vi "Set and Get Col Head String.vi"(7 "Mode":T1, 8 "错误输入":errorcluster, 10 "ColHdr Out In":string, 11 "Listbox Ref":refnum<vi>) -> (0 "错误输出":errorcluster, 2 "ColHdr Out":string, 3 "Dup Listbox Ref":refnum<vi>)   [LabVIEW 2012, in "Listbox Tool.lvlib"]
uses:
  Listbox Tool.lvlib
  Custom Type/Read and Write Mode.ctl
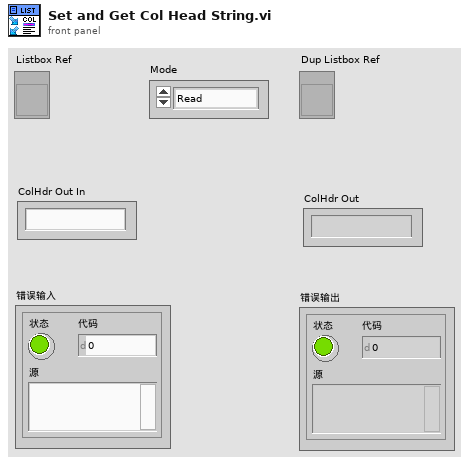
[diagram p1: front panel]
types:
  T1 = typedef "Listbox Tool.lvlib/Read and Write Mode.ctl" = enum16{"Read", "Write"}
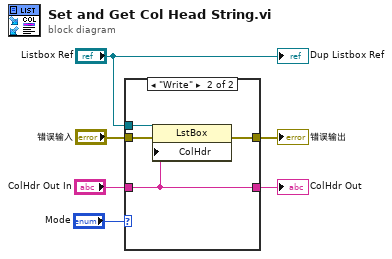
[diagram p0: block diagram]
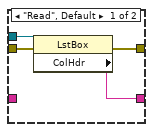
[diagram p2: hidden frame]
diagram:
  n1 = case shown="\"Write\"" "Mode" {
    tunnel: "ColHdr Out In" -> [_ w14]
    tunnel: [w10 w14] -> w4
    tunnel: "错误输入" -> [w8 w13]
    tunnel: "Listbox Ref" -> [w9 w12]
    tunnel: [w7 w11] -> w2
    frame "Read", Default {
      n2 = property class="LstBox"(reference=w9, error in=w8) -> (error out=w7:errorcluster, "ColHdr"=w10:string)  [unwired: 1 out]
    }
    frame "Write" {
      n3 = property class="LstBox"(reference=w12, error in=w13, "ColHdr"=w14) -> (error out=w11:errorcluster)  [unwired: 1 out]
    }
  }
  "错误输出" <- w2
  "ColHdr Out" <- w4
  "Dup Listbox Ref" <- "Listbox Ref"
